vi "daqmx_digital_1ch2linesboolean.vi"() -> ()   [LabVIEW 2019]
uses:
  <vilib>/DAQmx/read.llb/DAQmx Read (Digital 1D Bool 1Chan 1Samp).vi
  <vilib>/DAQmx/create/channels.llb/DAQmx Create Channel (DI-Digital Input).vi
  <vilib>/DAQmx/configure/task.llb/DAQmx Configure Logging (TDMS).vi
  <vilib>/DAQmx/miscellaneous.llb/DAQmx Fill In Error Info.vi
panel:
  in  "DAQmx Physical Channel":tag="PXI1Slot7/port0/line0:1"
  out "Error Out":errorcluster
  in  "TDMS File":path=path "C:/Python/projects/nitdms/tests/tdms_files/daqmx_digital_1ch2linesboolean.tdms"
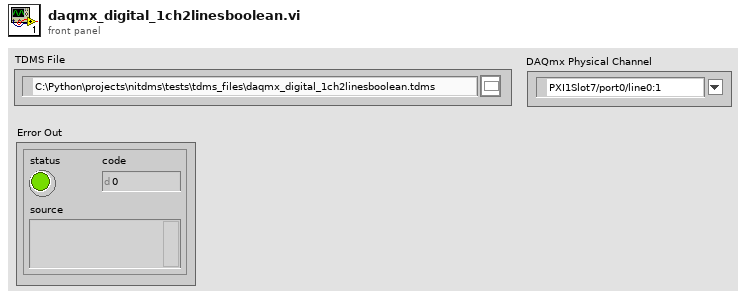
[diagram p1: front panel]
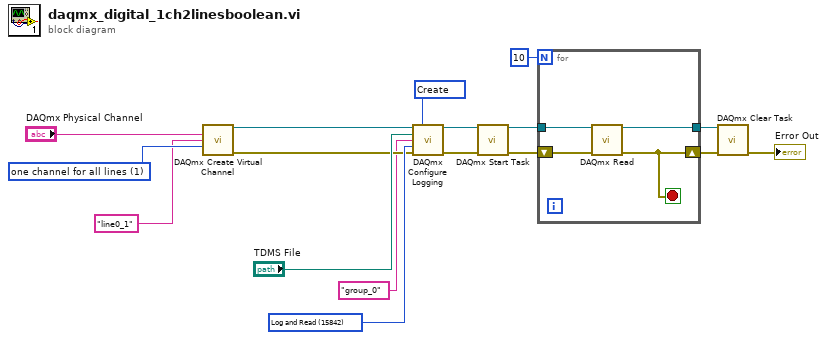
[diagram p0: block diagram]
diagram:
  w3 = 1 items=["one channel for each line", "one channel for all lines"] ("line grouping")
  w14 = 15842 items=["Off"=10231, "Log"=15844, "Log and Read"=15842] ("logging mode")
  w15 = 15848 items=["Open"=10437, "Open or Create"=15846, "Create or Replace"=15847, "Create"=15848] ("operation")
  n1 = call-poly <vilib>:"DAQmx Create Virtual Channel.vi"("lines"="DAQmx Physical Channel", "name to assign"="line0_1", "line grouping"=w3) -> ("task out"=w9:refnum<k21>, "error out"=w10:errorcluster)  [unwired: 11 in]
  n2 = call-poly <vilib>:"DAQmx Configure Logging.vi"("task/channels in"=w9, "operation"=w15, "file path"="TDMS File", "group name"="group_0", "logging mode"=w14, "error in"=w10) -> ("task out"=w12:refnum<k21>, "error out"=w13:errorcluster)  [unwired: 8 in]
  n3 = call <vilib>:"DAQmx Start Task.vi"("task/channels in"=w12, "error in"=w13) -> ("task out"=w7:refnum<k21>, "error out"=w8:errorcluster)  [unwired: 12 in]
  n4 = for {
    N: 10 -> [_]
    shift-right: [w18] -> w6
    shift-left: w8 -> [w21]
    tunnel: w7 -> [w20]
    tunnel: [w19] -> w4
    stop <- w18 stop-if-true
    n5 = call-poly <vilib>:"DAQmx Read.vi"("task/channels in"=w20, "error in"=w21) -> ("task out"=w19:refnum<k21>, "error out"=w18:errorcluster)  [unwired: 11 in, 1 out]
  }
  n6 = call <vilib>:"DAQmx Clear Task.vi"("task in"=w4, "error in"=w6) -> ("error out"=→"Error Out":errorcluster)  [unwired: 13 in]
